vi "Get Current Position.vi"(8 "error in (no error)":errorcluster, 11 "VISA resource name":refnum<visa-resource-name>) -> (0 "error out":errorcluster, 2 "Current Position out":u32, 3 "VISA resource name out":refnum<visa-resource-name>)   [LabVIEW 2018]
doc: "Retrieves the current position of the actuator.\n\n\n(Nimble Focus Consulting 2019)"
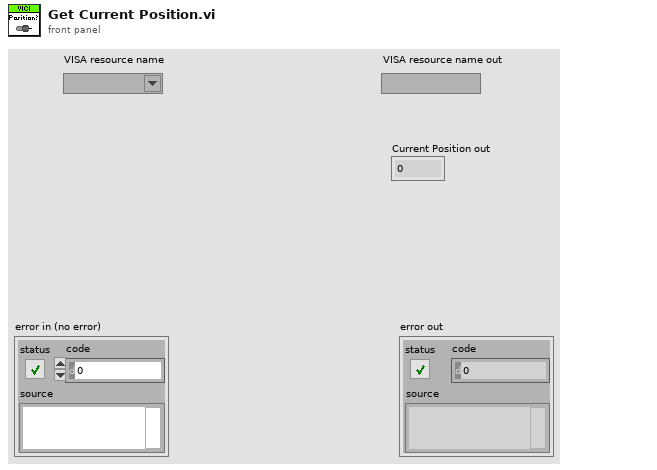
[diagram p1: front panel]
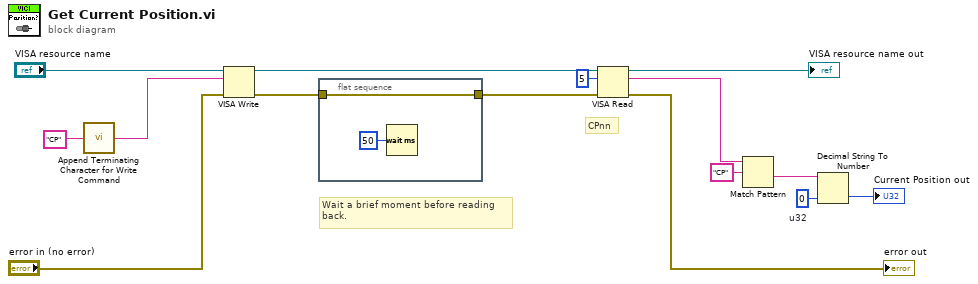
[diagram p0: block diagram]
diagram:
  w2 = u32 0  # u32
  # "Wait a brief moment before reading\nback."
  # "CPnn"
  n1 = call "Append Terminating Character for Write Command.vi"("Command in"="CP") -> ("Command with Terminating character out"=w13:string)
  n2 = VISA Write(VISA resource name="VISA resource name", write buffer=w13, error in (no error)="error in (no error)") -> (VISA resource name out=w9:refnum<visa-resource-name>, error out=w11:errorcluster)  [unwired: 1 out]
  n3 = flat-sequence {
    tunnel: w11 -> [w16]
    tunnel: [w16] -> w10
    frame #0 {
      n4 = Wait (ms)(milliseconds to wait=u32 50) -> ()  [unwired: 1 out]
    }
  }
  n5 = VISA Read(VISA resource name=w9, byte count=u32 5, error in (no error)=w10) -> (VISA resource name out=→"VISA resource name out":refnum<visa-resource-name>, read buffer=w6:string, error out=→"error out":errorcluster)  [unwired: 1 out]
  n6 = Match Pattern(string=w6, regular expression="CP") -> (after substring=w4:string)  [unwired: 1 in, 3 out]
  n7 = Decimal String To Number(string=w4, default (0L)=w2) -> (number=→"Current Position out":u32)  [unwired: 1 in, 1 out]
